vi "Circular_Buffer_Array.vi"(8 "Error In":errorcluster, 11 "Array":dbl[](array[numeric])) -> (0 "Error Out":errorcluster, 3 "output array":dbl[][](array[numeric])=[[4.0, 4.0, 4.0, 4.0, 4.0, 4.0, 4.0, 4.0, 4.0, 4.0, 4.0, 4.0, 4.0, 4.0, 4.0, 4.0, 4.0, 4.0, 4.0, 4.0]])   [LabVIEW 2014]
uses:
  Controls/FGVisfileopen.ctl
panel:
  out "s? t:f":i32
  in  "Input":dbl
  # "Circular Buffer"
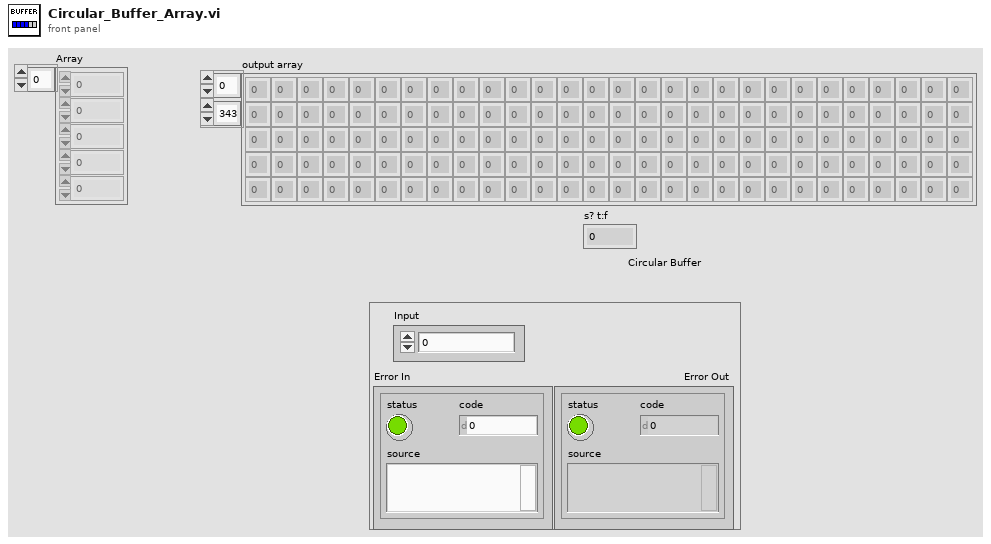
[diagram p1: front panel]
types:
  T1 = typedef "FGVisfileopen.ctl" = enum16{"Read", "Write"}
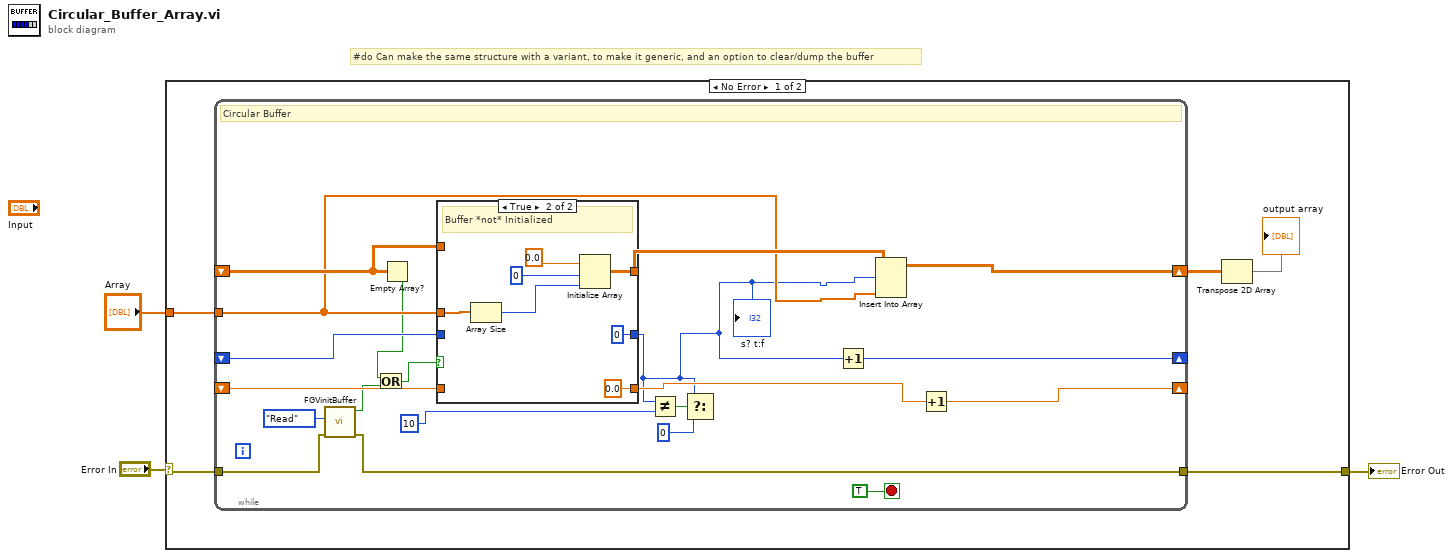
[diagram p0: block diagram]
diagram:
  # "#do Can make the same structure with a variant, to make it generic, and an option to clear/dump the buffer"
  n1 = case shown="No Error" "Error In" {
    selector: "Error In" -> [w8 w39]
    tunnel: [w7 w39] -> w2
    tunnel: "Array" -> [w6 _]
    frame No Error {
      n2 = while {
        tunnel: [w9] -> w7
        tunnel: w8 -> [w10]
        shift-right: [w16] -> _
        shift-left: _ -> [w21]
        shift-right: [w23] -> w5
        shift-left: _ -> [w28]
        tunnel: w6 -> [w22]
        shift-right: [w19] -> _
        shift-left: _ -> [w18]
        stop <- TRUE stop-if-true
        # "Circular Buffer"
        n3 = call "FGVinitBuffer.vi"("error in"=w10, "Write/Read?"=FGVisfileopen."Read" ("Write from FGV or Read from FGV?")) -> ("error out"=w9:errorcluster, "Output Value"=w13:bool)  [unwired: 8 in]
        n4 = Empty Array?(array=w28) -> (empty?=w12:bool)
        n5 = Or(x=w12, y=w13) -> (x .or. y?=w11:bool)
        n6 = case shown="True" w11 {
          tunnel: [w30 0] -> w15
          tunnel: w21 -> [w30 _]
          tunnel: [w31 w34] -> w24
          tunnel: w28 -> [w31 _]
          tunnel: w22 -> [_ w36]
          tunnel: w18 -> [w29 _]
          tunnel: [w29 0.0] -> w17
          frame False {
            # "Buffer was already Initialized"
          }
          frame True {
            # "Buffer *not* Initialized"
            n7 = Array Size(array=w36) -> (size(s)=w35:i32)
            n8 = Initialize Array(0.0 ("element"), 0 ("dimension size"), w35) -> (w34:dbl[][])
          }
        }
        "s? t:f" <- w15
        n9 = Not Equal?(x=w15, y=10) -> (x != y?=w27:bool)
        n10 = Select(t=w15, s=w27, f=0) -> ()  [unwired: 1 out]
        n11 = Increment(x=w15) -> (x+1=w16:i32)
        n12 = Insert Into Array(array=w24, index (row)=w15, new element=w22) -> (w23:dbl[][])  [unwired: 1 in]
        n13 = Increment(x=w17) -> (x+1=w19:dbl)
      }
      n14 = Transpose 2D Array(2D array=w5) -> (transposed array=→"output array":dbl[][])
    }
    frame Error {
    }
  }
  "Error Out" <- w2
